vi "Average 2D Array.vi"(11 "Image Pixels (U8)":u8[][](array[numeric])) -> (3 "Numeric":dbl)   [LabVIEW 2014]
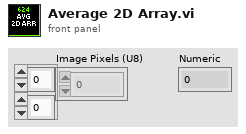
[diagram p1: front panel]
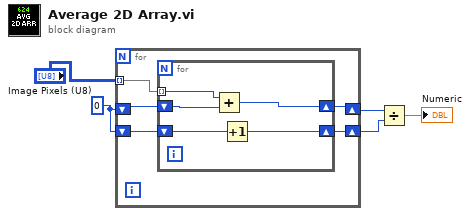
[diagram p0: block diagram]
diagram:
  w2 = 0
  n1 = for {
    tunnel: "Image Pixels (U8)" -> [w10] mode=indexing
    shift-right: [w9] -> w3
    shift-left: w2 -> [w8]
    shift-right: [w6] -> w4
    shift-left: w2 -> [w7]
    n2 = for {
      tunnel: w10 -> [w15] mode=indexing
      shift-right: [w14] -> w9
      shift-left: w8 -> [w13]
      shift-right: [w11] -> w6
      shift-left: w7 -> [w12]
      n3 = Add(x=w15, y=w13) -> (x+y=w14:i32)
      n4 = Increment(x=w12) -> (x+1=w11:i32)
    }
  }
  n5 = Divide(x=w3, y=w4) -> (x/y=→"Numeric":dbl)
